vi "ProvisioningVerifyVersionsResponse_Create.vi"(7 "Header":T2, 8 "error in (no error)":errorcluster, 9 "ResponseError":errorcluster, 11 "IRoutingSource":T1) -> (0 "error out":errorcluster, 3 "Message":T4)   [LabVIEW 2017]
uses:
  <vilib>/addons/InsightCM/MessageBus/Base/controls/Message.ctl
  <vilib>/addons/InsightCM/MessageBus/Base/controls/MessageHeader.ctl
  <vilib>/addons/InsightCM/MessageBus/Base/controls/KeyValuePair.ctl
  <vilib>/addons/InsightCM/MessageBus/Base/controls/IRoutingSource.ctl
  <vilib>/addons/InsightCM/MessageBus/Base/controls/MessageClassType.ctl
  <vilib>/addons/InsightCM/Utilities/PropertyHelpers/PropertyHelpers.lvlib
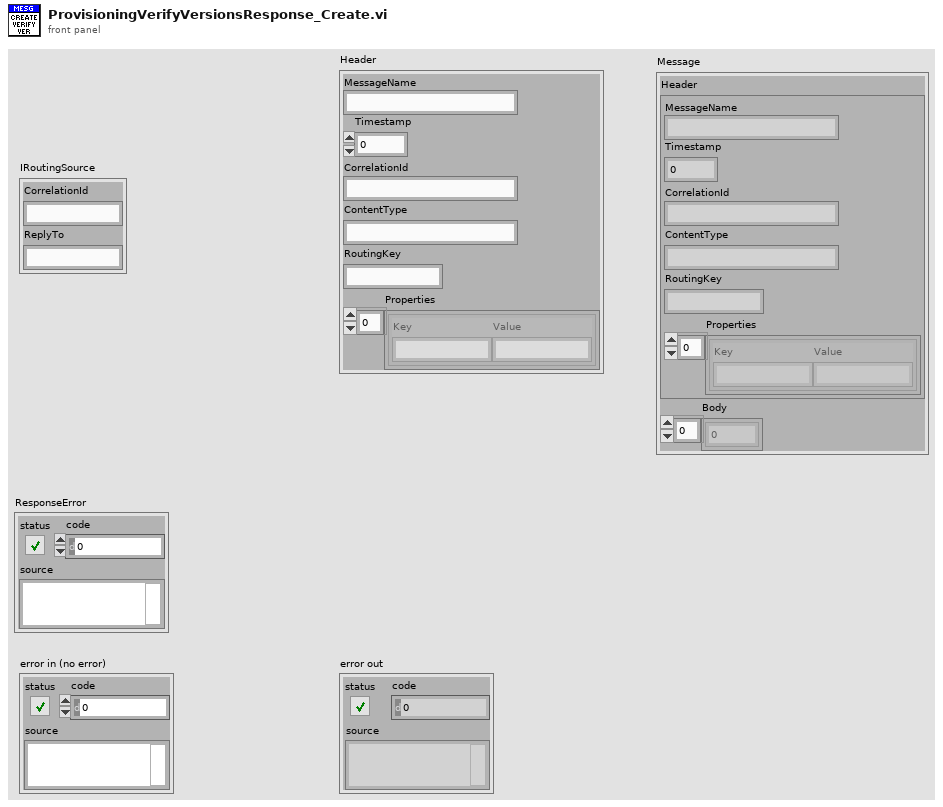
[diagram p1: front panel]
types:
  T1 = typedef "IRoutingSource.ctl" = cluster{"CorrelationId":string, "ReplyTo":string}
  T2 = typedef "MessageHeader.ctl" = cluster{"MessageName":string, "Timestamp":i64, "CorrelationId":string, "ContentType":string, "RoutingKey":string, "Properties":T3[]}
  T3 = typedef "KeyValuePair.ctl" = cluster{"Key":string, "Value":string}
  T4 = typedef "Message.ctl" = cluster{"Header":T2, "Body":u8[]}
  T5 = typedef "MessageClassType.ctl" = enum16{"Request", "Response", "Broadcast", "RoutedMessage"}
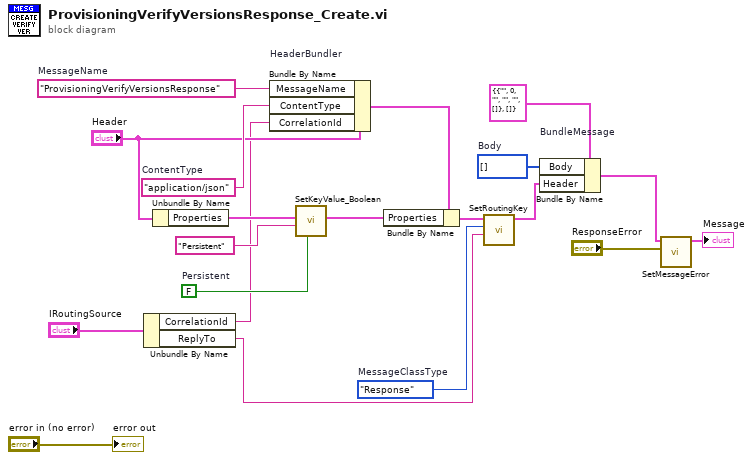
[diagram p0: block diagram]
diagram:
  w19 = u8[] []  # Body
  w17 = MessageClassType."Response"  # MessageClassType
  w12 = FALSE  # Persistent
  w18 = "ProvisioningVerifyVersionsResponse"  # MessageName
  w15 = "application/json"  # ContentType
  n1 = Unbundle By Name("IRoutingSource") -> ("CorrelationId"=w2:string, "ReplyTo"=w1:string)
  n2 = Unbundle By Name("Header") -> ("Properties"=w14:T3[])
  n3 = Bundle By Name "HeaderBundler"(cluster="Header", "MessageName"=w18, "ContentType"=w15, "CorrelationId"=w2) -> (w9:T2)
  n4 = call <vilib>:"SetKeyValue_Boolean.vi"("value"=w12, "key"="Persistent" ("Key"), "key value pairs"=w14) -> ("key value pairs out"=w8:T3[])  [unwired: 8 in]
  n5 = Bundle By Name(cluster=w9, "Properties"=w8) -> (w10:T2)
  n6 = call <vilib>:"SetRoutingKey.vi"("SendTo"=w1, "MessageClassType"=w17, "Message Header in"=w10) -> ("Message Header out"=w11:T2)  [unwired: 8 in]
  n7 = Bundle By Name "BundleMessage"(cluster=T4 {"Header"={"MessageName"="", "Timestamp"=0, "CorrelationId"="", "ContentType"="", "RoutingKey"="", "Properties"=[]}, "Body"=[]} ("Message"), "Body"=w19, "Header"=w11) -> (w6:T4)
  n8 = call <vilib>:"SetMessageError.vi"("error"="ResponseError", "message in"=w6) -> ("message out"=→"Message":T4)  [unwired: 9 in]
  "error out" <- "error in (no error)"
